vi "control motor a pasos.vi"() -> ()   [LabVIEW 2012]
uses:
  <vilib>/LabVIEW Interface for Arduino/Type Defs/Board Type.ctl
  <vilib>/LabVIEW Interface for Arduino/LabVIEW Interface for Arduino.lvlib
panel:
  in  "Set Acceleration (0 to disable)":i16
  in  "pasos":i16
  in  "velocidad":i16=100
  in  "stop":bool
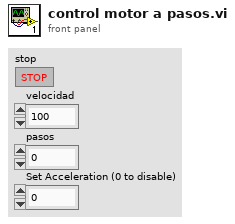
[diagram p1: front panel]
types:
  T1 = typedef "LabVIEW Interface for Arduino.lvlib/Board Type.ctl" = enum16{"Uno", "Dimuelanove w/Atmega 328", "Mega 2560"}
  T2 = typedef "LabVIEW Interface for Arduino.lvlib/Arduino Resource.ctl" = cluster{"VISA resource":refnum<visa-resource-name>, "Board Type":T1, "Connection Type":enum8{"USB / Serial"}, "Bytes Per Packet (15)":u8}
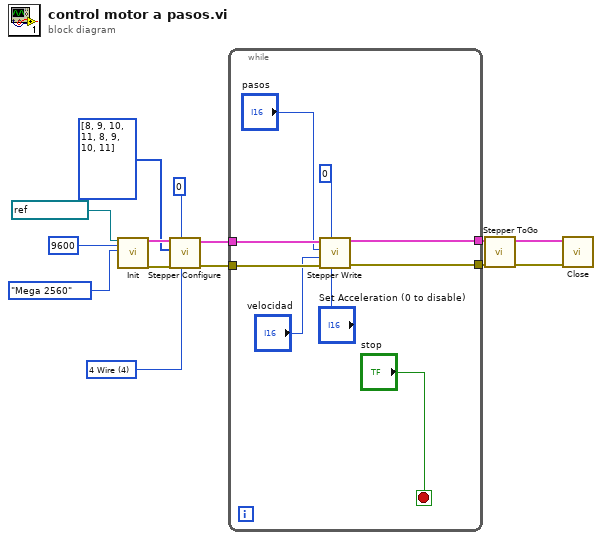
[diagram p0: block diagram]
diagram:
  w10 = u8 4 items=["2 Wire (Pulse & Direction)"=1, "2 Wire"=2, "4 Wire"=4, "EasyDriver"=6, "AF Motor Shield (Stepper 1 & 2 Only)"=5] ("Control Method")
  n1 = call <vilib>:"Init.vi"("VISA resource"=refnum<visa-resource-name> "COM7", "Baud Rate (115200)"=u32 9600, "Board Type (Uno)"=Board_Type."Mega 2560") -> ("Arduino Resource"=w11:T2, "error out"=w12:errorcluster)  [unwired: 15 in]
  n2 = call <vilib>:"Stepper Configure.vi"("Control Method"=w10, "Stepper #"=u8 0, "error in"=w12, "Stepper Pins"=u8[] [8, 9, 10, 11, 8, 9, 10, 11], "Arduino Resource"=w11) -> ("error out"=w7:errorcluster, "Arduino Resource Out"=w8:T2)  [unwired: 5 in]
  n3 = while {
    tunnel: w8 -> [w22]
    tunnel: w7 -> [w21]
    tunnel: [w18] -> w6
    tunnel: [w17] -> w5
    stop <- "stop" stop-if-true
    n4 = call <vilib>:"Stepper Write.vi"("Set Acceleration (0 to disable)"="Set Acceleration (0 to disable)", "Stepper #"=u8 0, "error in"=w21, "Set Speed (Steps per Second)"="velocidad", "# of Steps to Move"="pasos", "Arduino Resource"=w22) -> ("error out"=w17:errorcluster, "Arduino Resource Out"=w18:T2)  [unwired: 4 in]
  }
  n5 = call <vilib>:"Stepper ToGo.vi"("error in"=w5, "Arduino Resource"=w6) -> ("error out"=w3:errorcluster, "Arduino Resource Out"=w4:T2)  [unwired: 6 in, 2 out]
  n6 = call <vilib>:"Close.vi"("Arduino Resource"=w4, "error in"=w3) -> ()  [unwired: 13 in, 1 out]
